vi "FGV Variant.vi"(9 "Data":variant, 10 "name":string, 11 "Function":enum16{"Reset data", "Get data", "Set data"}(ring)) -> (1 "found?":bool, 2 "replaced?":bool, 3 "value":variant)   [LabVIEW 2020]
doc: "Variable global funcional para guardar y obtener datos"
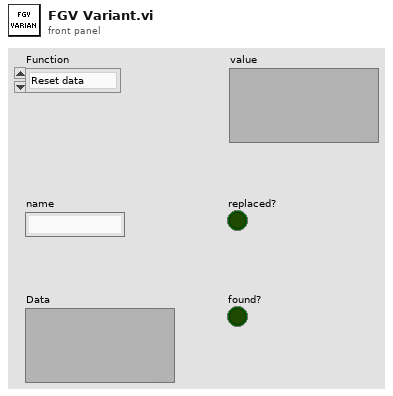
[diagram p1: front panel]
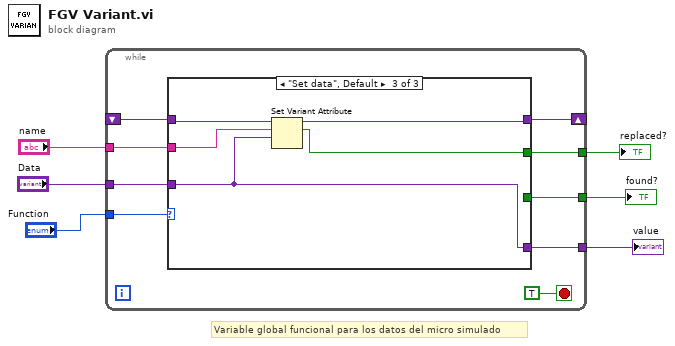
[diagram p0: block diagram]
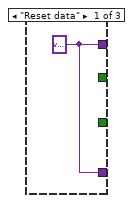
[diagram p2: hidden frame]
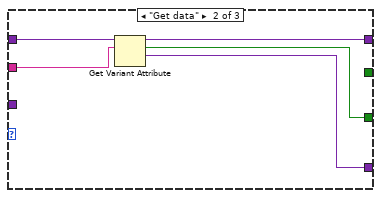
[diagram p3: hidden frame]
diagram:
  # "Variable global funcional para los datos del micro simulado"
  n1 = while {
    tunnel: "Function" -> [w15]
    shift-right: [w14] -> _
    shift-left: _ -> [w13]
    tunnel: "name" -> [w11]
    tunnel: "Data" -> [w10]
    tunnel: [w9] -> w3
    tunnel: [w8] -> w2
    tunnel: [w7] -> w1
    stop <- TRUE stop-if-true
    n2 = case shown="\"Set data\", Default" w15 {
      tunnel: [w16 w19 w25] -> w14
      tunnel: w13 -> [_ w21 w26]
      tunnel: w11 -> [_ w20 w24]
      tunnel: w10 -> [_ _ w22]
      tunnel: [_ _ w23] -> w9
      tunnel: [_ w18 _] -> w8
      tunnel: [w16 w17 w22] -> w7
      frame "Reset data" {
        w16 = variant
      }
      frame "Get data" {
        n3 = Get Variant Attribute(Variant=w21, name=w20) -> (duplicate Variant=w19:variant, found=w18:bool, value=w17:variant)  [unwired: 2 in, 1 out]
      }
      frame "Set data", Default {
        n4 = Set Variant Attribute(Variant=w26, name=w24, value=w22) -> (Variant out=w25:variant, replaced=w23:bool)  [unwired: 1 in, 1 out]
      }
    }
  }
  "replaced?" <- w3
  "found?" <- w2
  "value" <- w1
